vi "Hausmodell.Bodentemperatur.vi"(6 "Error IN":errorcluster, 9 "Hausmodell IN":refnum<data-value>) -> (0 "Error OUT":errorcluster, 3 "Hausmodell OUT":refnum<data-value>)   [LabVIEW 2016, in "Hausmodell.lvclass"]
uses:
  Hausmodell.lvclass
  Hausmodell.lvclass/Hausmodell.ctl
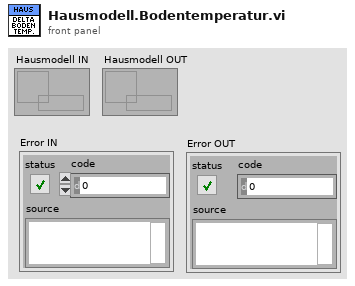
[diagram p1: front panel]
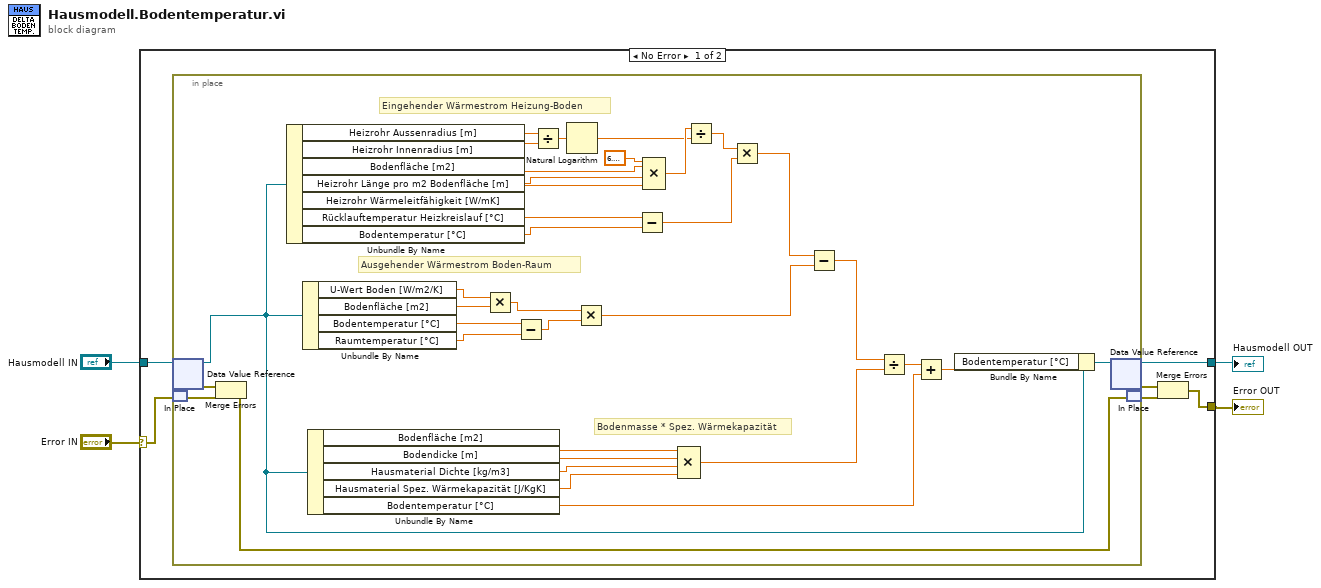
[diagram p0: block diagram]
diagram:
  n1 = case shown="No Error" "Error IN" {
    selector: "Error IN" -> [w9 w47]
    tunnel: [w10 w46] -> w3
    tunnel: [w7 w47] -> w1
    tunnel: "Hausmodell IN" -> [w5 w46]
    frame No Error {
      n2 = in-place {
        # "Bodenmasse * Spez. Wärmekapazität"
        # "Ausgehender Wärmestrom Boden-Raum"
        # "Eingehender Wärmestrom Heizung-Boden"
        n3 = in-place-dvr #1(w5) -> (w15:refnum<class "Hausmodell.lvclass">, w45:errorcluster)
        n4 = in-place-match #2(w9) -> (w44:errorcluster)
        n5 = Merge Errors(w45, w44) -> (w13:errorcluster)
        n6 = Unbundle By Name(w15) -> ("Heizrohr Aussenradius [m]"=w20:dbl, "Heizrohr Innenradius [m]"=w19:dbl, "Bodenfläche [m2]"=w18:dbl, "Heizrohr Länge pro m2 Bodenfläche [m]"=w17:dbl, "Heizrohr Wärmeleitfähigkeit [W/mK]"=w16:dbl, "Rücklauftemperatur Heizkreislauf [°C]"=w12:dbl, "Bodentemperatur [°C]"=w11:dbl)
        n7 = Unbundle By Name(w15) -> ("U-Wert Boden [W/m2/K]"=w24:dbl, "Bodenfläche [m2]"=w23:dbl, "Bodentemperatur [°C]"=w22:dbl, "Raumtemperatur [°C]"=w21:dbl)
        n8 = Unbundle By Name(w15) -> ("Bodenfläche [m2]"=w29:dbl, "Bodendicke [m]"=w28:dbl, "Hausmaterial Dichte [kg/m3]"=w27:dbl, "Hausmaterial Spez. Wärmekapazität [J/KgK]"=w26:dbl, "Bodentemperatur [°C]"=w25:dbl)
        n9 = Multiply(x=w24, y=w23) -> (x*y=w39:dbl)
        n10 = Subtract(x=w22, y=w21) -> (x-y=w38:dbl)
        n11 = Divide(x=w20, y=w19) -> (x/y=w35:dbl)
        n12 = Natural Logarithm(1:w35) -> (0:w31:dbl)
        n13 = Multiply(x=w39, y=w38) -> (x*y=w37:dbl)
        n14 = Subtract(x=w12, y=w11) -> (x-y=w30:dbl)
        n15 = Compound Arithmetic op=MULTIPLY(6.283185307179586, w18, w17, w16) -> (w32:dbl)
        n16 = Compound Arithmetic op=MULTIPLY(w29, w28, w27, w26) -> (w36:dbl)
        n17 = Divide(x=w32, y=w31) -> (x/y=w33:dbl)
        n18 = Multiply(x=w33, y=w30) -> (x*y=w43:dbl)
        n19 = Subtract(x=w43, y=w37) -> (x-y=w42:dbl)
        n20 = Divide(x=w42, y=w36) -> (x/y=w41:dbl)
        n21 = Add(x=w41, y=w25) -> (x+y=w40:dbl)
        n22 = Bundle By Name(cluster=w15, "Bodentemperatur [°C]"=w40) -> (w14:refnum<class "Hausmodell.lvclass">)
        n23 = in-place-dvr #1(w14) -> (w10:refnum<data-value>, w8:errorcluster)
        n24 = in-place-match #2(w13) -> (w6:errorcluster)
      }
      n25 = Merge Errors(w8, w6) -> (w7:errorcluster)
    }
    frame Error {
    }
  }
  "Hausmodell OUT" <- w3
  "Error OUT" <- w1
